vi "Unflatten Value.vi"(8 "Error In":errorcluster, 10 "Value":string, 11 "String In":refnum<class "String.lvclass">) -> (0 "Error Out":errorcluster, 3 "String Out":refnum<class "String.lvclass">)   [LabVIEW 2017, in "Tree API.lvlib" / "String.lvclass"]
uses:
  String.lvclass
  Tree Manager/Tree.lvclass
  <vilib>/regexp/Match Regular Expression.xnode
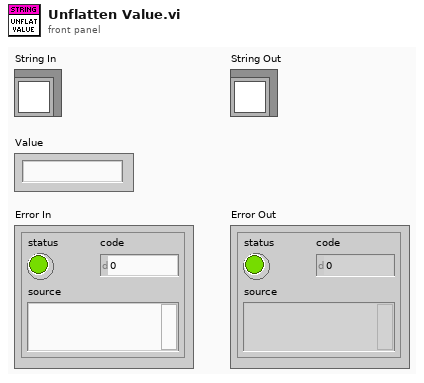
[diagram p1: front panel]
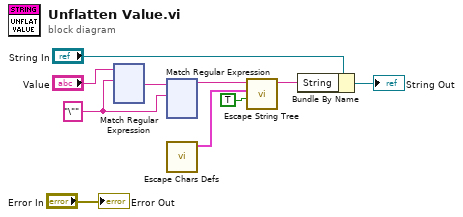
[diagram p0: block diagram]
diagram:
  w5 = "\"" ("regular expression")
  n1 = xnode "Match Regular Expression"("input string"="Value", "regular expression"=w5) -> ("after match"=w6:string)  [unwired: 4 in, 4 out]
  n2 = xnode "Match Regular Expression"("input string"=w6, "regular expression"=w5) -> ("before match"=w4:string)  [unwired: 4 in, 4 out]
  n3 = call "Escape Chars Defs.vi"() -> ("Escapes"=w3:cluster{"String":string, "Escape":string}[])  [unwired: 11 in]
  n4 = call "Escape String Tree.vi"("Reverse? (False)"=TRUE ("Remove Escapes? (False)"), "Escapes"=w3, "String In"=w4) -> ("String Out"=w1:string)  [unwired: 8 in]
  n5 = Bundle By Name(cluster="String In", "String"=w1) -> (→"String Out":refnum<class "String.lvclass">)
  "Error Out" <- "Error In"
